vi "Excel Disable Precision as Displayed.vi"(8 "error in (no error)":errorcluster, 11 "report in":refnum<class "NI_report.lvclass">) -> (0 "error out":errorcluster, 3 "report out":refnum<class "NI_report.lvclass">)   [LabVIEW 2020, in "varilib.lvlib"]
doc: "Disables 'Precision as Displayed' in the current opened Excel file. This terrible excel feature can cause loss of data, therefore this vi disables it. Use it right after opening an Excel file."
uses:
  varilib.lvlib
  <vilib>/Utility/NIReport.llb/Excel/NI_Excel.lvclass
  <vilib>/Utility/NIReport.llb/NI_report.lvclass
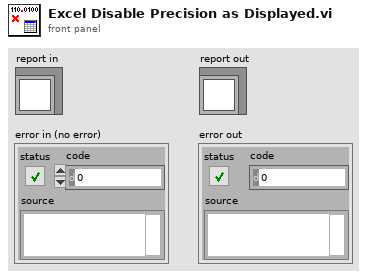
[diagram p1: front panel]
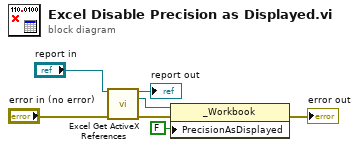
[diagram p0: block diagram]
diagram:
  n1 = call <vilib>:"Excel Get ActiveX References.vi"("report in"="report in", "error in (no error)"="error in (no error)") -> ("report out"=→"report out":refnum<class "NI_report.lvclass">, "Excel._Workbook"=w1:refnum<k7>, "error out"=w2:errorcluster)  [unwired: 7 in, 4 out]
  n2 = property class="_Workbook"(reference=w1, error in=w2, "PrecisionAsDisplayed"=FALSE) -> (error out=→"error out":errorcluster)  [unwired: 1 out]
